vi "test Write.vi"(11 "Test Case In":refnum<class "Test PCANBasic.lvclass">) -> (0 "error out":errorcluster, 3 "Test Case Out":refnum<class "Test PCANBasic.lvclass">)   [LabVIEW 2020, in "Test PCANBasic.lvclass"]
uses:
  Test PCANBasic.lvclass
  C:/Program Files/National Instruments/LabVIEW 2026/vi.lib/Astemes/LUnit/Test Case.lvclass
  <vilib>/Astemes/LUnit/Test Case.lvclass/Test Case.ctl
  source/PCANBasic.lvlib
  <vilib>/Astemes/LUnit/Test Case.lvclass
  Global PCAN Channel.vi
  Global PCAN Baudrate.vi
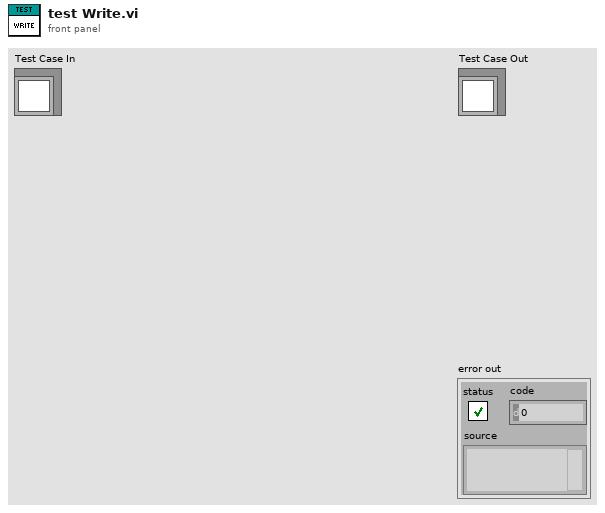
[diagram p1: front panel]
types:
  T1 = cluster{"ID":u32, "MSGTYPE":cluster{"Type":u8, "Extended":bool, "Echo":bool}, "LEN":u8, "DATA":cluster{"0":u8, "1":u8, "2":u8, "3":u8, "4":u8, "5":u8, "6":u8, "7":u8}}
  T2 = cluster{"0":u8, "1":u8, "2":u8, "3":u8, "4":u8, "5":u8, "6":u8, "7":u8}
  T3 = typedef "PCANBasic.lvlib/PCAN Baud.ctl" = u16
  T4 = typedef "PCANBasic.lvlib/TPCANHandle.ctl" = u16
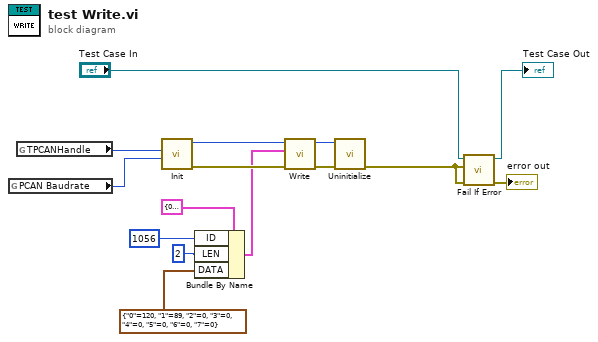
[diagram p0: block diagram]
diagram:
  n1 = global read "Global PCAN Baudrate.vi" "PCAN Baudrate"() -> (w12:T3)
  n2 = global read "Global PCAN Channel.vi" "TPCANHandle"() -> (w11:T4)
  n3 = call "Init.vi"("Baudrate"=w12, "Channel"=w11) -> ("error out"=w10:errorcluster, "TPCANHandle out"=w8:T4)  [unwired: 7 in, 1 out]
  n4 = Bundle By Name(cluster=T1 {"ID"=0, "MSGTYPE"={"Type"=0, "Extended"=FALSE, "Echo"=FALSE}, "LEN"=0, "DATA"={"0"=0, "1"=0, "2"=0, "3"=0, "4"=0, "5"=0, "6"=0, "7"=0}} ("PCAN Message"), "ID"=u32 1056, "LEN"=u8 2, "DATA"=T2 {"0"=120, "1"=89, "2"=0, "3"=0, "4"=0, "5"=0, "6"=0, "7"=0}) -> (w1:T1)
  n5 = call "Write.vi"("error in"=w10, "PCAN Message"=w1, "TPCANHandle in"=w8) -> ("error out"=w9:errorcluster, "TPCANHandle out"=w7:T4)  [unwired: 6 in, 1 out]
  n6 = call "Uninitialize.vi"("error in"=w9, "TPCANHandle in"=w7) -> ("error out"=w3:errorcluster)  [unwired: 8 in, 1 out]
  n7 = call <vilib>:"Fail If Error.vi"("error in (no error)"=w3, "Assert error"=w3, "LUnit Test Case In"="Test Case In") -> ("error out"=→"error out":errorcluster, "LUnit Test Case Out"=→"Test Case Out":refnum<class "Test PCANBasic.lvclass">)  [unwired: 7 in]
